vi "Square Colors.vi"(11 "Game in":refnum<class "Game.lvclass">) -> (2 "Square Colors":u32[][](array[colorbox]), 3 "Game out":refnum<class "Game.lvclass">)   [LabVIEW 2020, in "SquareBattle.lvlib" / "Game.lvclass"]
uses:
  Game.lvclass
  Game.lvclass/Game.ctl
  Map/Map.lvclass
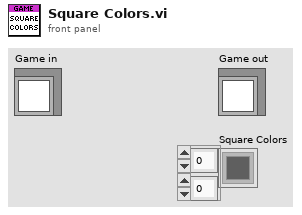
[diagram p1: front panel]
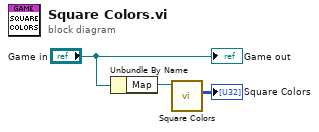
[diagram p0: block diagram]
diagram:
  n1 = Unbundle By Name("Game in") -> ("Map"=w2:refnum<class "Map.lvclass">)
  n2 = call "Square Colors.vi"("Map in"=w2) -> ("Square Colors"=→"Square Colors":u32[][])  [unwired: 9 in, 1 out]
  "Game out" <- "Game in"
